vi "SendData.vi"(0 "reference":refnum<class "VdRs232.lvclass">, 1 "charactersToWrite":string, 5 "error in (no error)":errorcluster, 6 "WaitForOtherProcessesToBeFinished(True)":bool=TRUE) -> (14 "duplicate reference":refnum<class "VdRs232.lvclass">, 15 "charsWritten":u32, 19 "error out":errorcluster)   [LabVIEW 2020, in "VdRs232.lvclass"]
doc: "Tansmits data on the com-port"
uses:
  VdRs232.lvclass
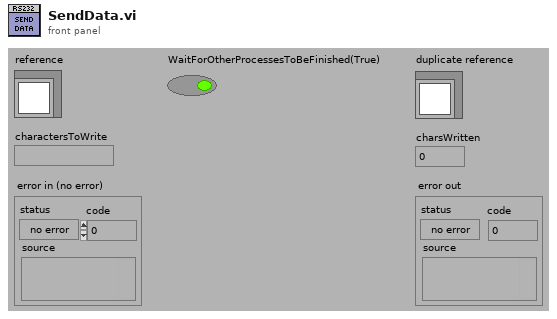
[diagram p1: front panel]
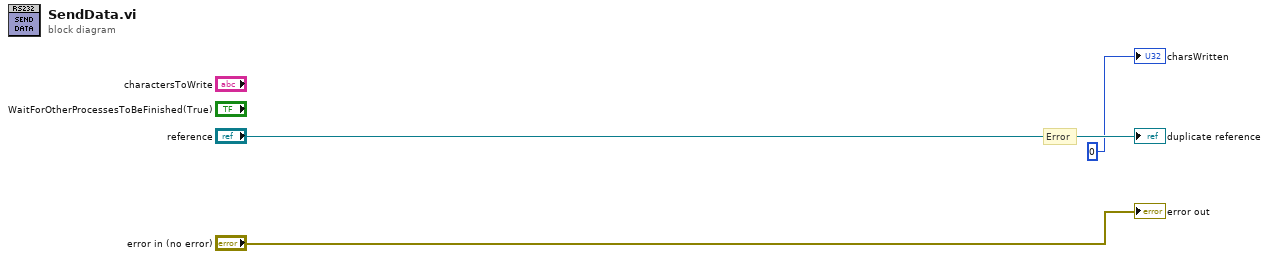
[diagram p0: block diagram]
diagram:
  # "Error"
  "error out" <- "error in (no error)"
  "duplicate reference" <- "reference"
  "charsWritten" <- u32 0 ("return count")
